vi "filepathsubvi.vi"(8 "error in (no error)":errorcluster, 10 "String":string, 11 "String 2":string) -> (0 "error out":errorcluster, 1 "actual path":path, 2 "Orignal Path":path, 3 "actual path 2":path, 5 "Path 2":path)   [LabVIEW 2017]
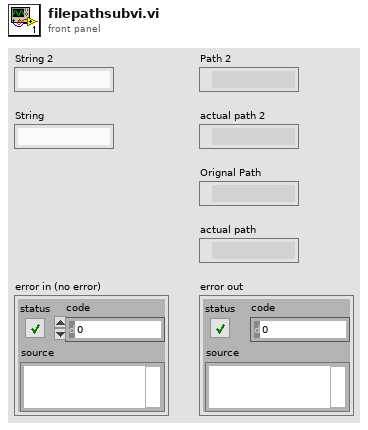
[diagram p1: front panel]
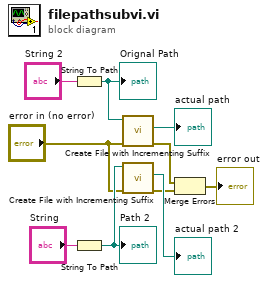
[diagram p0: block diagram]
diagram:
  n1 = String To Path(string="String 2") -> (path=w10:path)
  "Orignal Path" <- w10
  n2 = String To Path(string="String") -> (path=w8:path)
  "Path 2" <- w8
  n3 = call <vilib>:"Create File with Incrementing Suffix.vi"("error in (no error)"="error in (no error)", "file path"=w10) -> ("error out"=w3:errorcluster, "actual path"=→"actual path":path)  [unwired: 7 in, 1 out]
  n4 = call <vilib>:"Create File with Incrementing Suffix.vi"("error in (no error)"="error in (no error)", "file path"=w8) -> ("error out"=w4:errorcluster, "actual path"=→"actual path 2":path)  [unwired: 7 in, 1 out]
  n5 = Merge Errors(w3, w4) -> (→"error out":errorcluster)
